vi "Destroy Subpanel.vi"(7 "Skip Manager Close":bool, 8 "error in (no error)":errorcluster, 11 "CIF_UI in":refnum<class "CIF_UI.lvclass">) -> (0 "error out":errorcluster, 3 "CIF_UI out":refnum<class "CIF_UI.lvclass">)   [LabVIEW 2021, in "CIF_UI.lvclass"]
uses:
  CIF_UI.lvclass
  CIF_UI.lvclass/CIF_UI.ctl
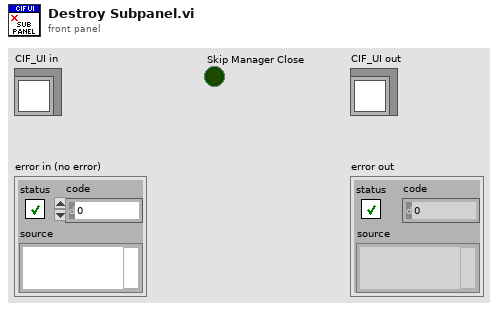
[diagram p1: front panel]
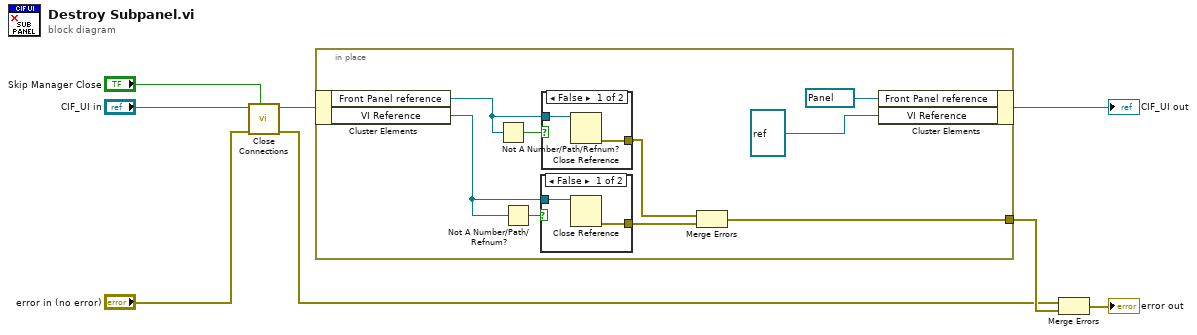
[diagram p0: block diagram]
diagram:
  n1 = call "Close Connections.vi"("Skip Manager Close"="Skip Manager Close", "error in (no error)"="error in (no error)", "CIF_UI in"="CIF_UI in") -> ("error out"=w5:errorcluster, "CIF_UI out"=w4:refnum<class "CIF_UI.lvclass">)  [unwired: 7 in]
  n2 = in-place {
    in-place-border: [w9] -> w7
    n3 = in-place-cluster #1(w4) -> ("Front Panel reference"=w14:refnum<vi>, "VI Reference"=w16:refnum<vi>)
    n4 = Not A Number/Path/Refnum?(number/path/refnum=w14) -> (NaN/Path/Refnum?=w15:bool)
    n5 = Not A Number/Path/Refnum?(number/path/refnum=w16) -> (NaN/Path/Refnum?=w17:bool)
    n6 = case shown="False" w17 {
      tunnel: w16 -> [w21 _]
      tunnel: [w20 _] -> w11
      frame False {
        n7 = Close Reference(reference=w21) -> (error out=w20:errorcluster)  [unwired: 1 in]
      }
      frame True {
      }
    }
    n8 = case shown="False" w15 {
      tunnel: w14 -> [w19 _]
      tunnel: [w18 _] -> w10
      frame False {
        n9 = Close Reference(reference=w19) -> (error out=w18:errorcluster)  [unwired: 1 in]
      }
      frame True {
      }
    }
    n10 = Merge Errors(w10, w11) -> (w9:errorcluster)
    n11 = in-place-cluster #1("Front Panel reference"=refnum<vi> refnum, "VI Reference"=refnum<vi> refnum) -> (→"CIF_UI out":refnum<class "CIF_UI.lvclass">)
  }
  n12 = Merge Errors(w5, w7) -> (→"error out":errorcluster)
